vi "Create an FPGA Addon and selectively import scalars.vi"() -> ()   [LabVIEW 2018]
uses:
  <vilib>/addons/VeriStand Custom Device Scripting APIs/FPGA Addon/Scripting API.lvlibp/APIs/Scripting API/TypeDefs/Output Scalar Data.ctl
  <vilib>/addons/VeriStand Custom Device Scripting APIs/FPGA Addon/Scripting API.lvlibp/Addon/Addon Shared/Types/Data Type.ctl
  <vilib>/addons/VeriStand Custom Device Scripting APIs/FPGA Addon/Scripting API.lvlibp/APIs/Scripting API/TypeDefs/Input Scalar Data.ctl
  <vilib>/addons/VeriStand Custom Device Scripting APIs/FPGA Addon/Scripting API.lvlibp/APIs/Scripting API/Public/Bitfile Resources/Import Bitfile Scalars (Instances)/Import Scalars - by label.vi
  <vilib>/addons/VeriStand Custom Device Scripting APIs/FPGA Addon/Scripting API.lvlibp
  <vilib>/addons/VeriStand Custom Device Scripting APIs/FPGA Addon/Scripting API.lvlibp/Addon/Addon Shared/FPGA Addon Shared.lvlib
panel:
  out "imported bitfile scalars out":T1[](array[typedef])
  out "error out":errorcluster
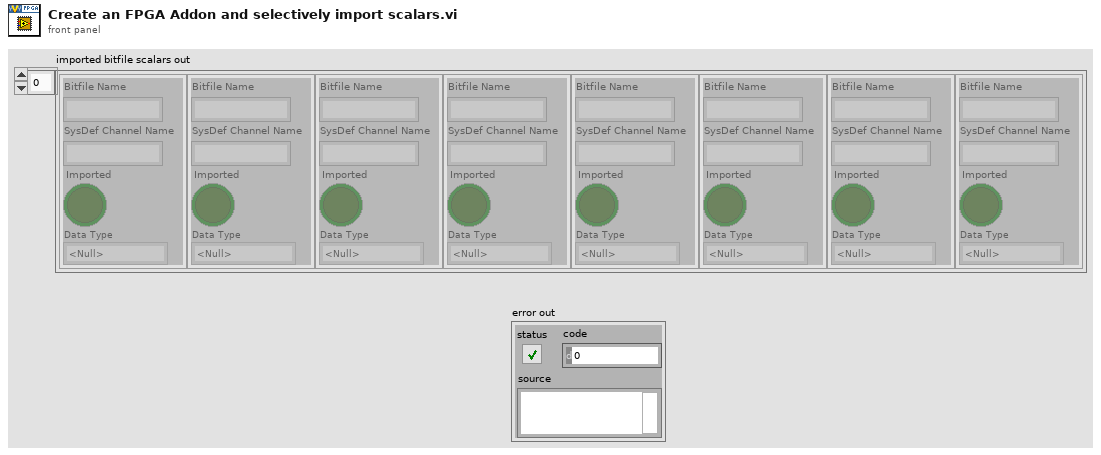
[diagram p1: front panel]
types:
  T1 = typedef "Scripting API.lvlibp/Output Scalar Data.ctl" = cluster{"Bitfile Name":string, "SysDef Channel Name":string, "Imported":bool, "Data Type":T2}
  T2 = typedef "Scripting API.lvlibp/FPGA Addon Shared.lvlib/Data Type.ctl" = enum8{"<Null>", "I8", "I16", "I32", "I64", "U8", "U16", "U32", "U64", "SGL", "Boolean", "Analog PWM In Settings", "Analog PWM In", "Digital PWM In Settings", "Digital PWM In", "Digital PWM Out", "Sine Out", "FXP+/-24.5", "FXP+/-16.5", "FXP+/-32.8", "FXP+/-64.32", "FXP+/-16.7", "FXP+/-20.5", "FXP+/-27.5", "FXP+/-32.16", "FXP+16.3", "FXP+18.3", "Digital Static In", "Digital Static Out", "Digital Static In Settings", "Digital WSS Out", "Quad Encoder Settings", "Quad Encoder In", "Group"}
  T3 = typedef "Scripting API.lvlibp/Input Scalar Data.ctl" = cluster{"Bitfile Name":string, "SysDef Name":string}
  T4 = typedef "Scripting API.lvlibp/Custom Device API.lvlib/Custom Device Item Ref.ctl" = u64
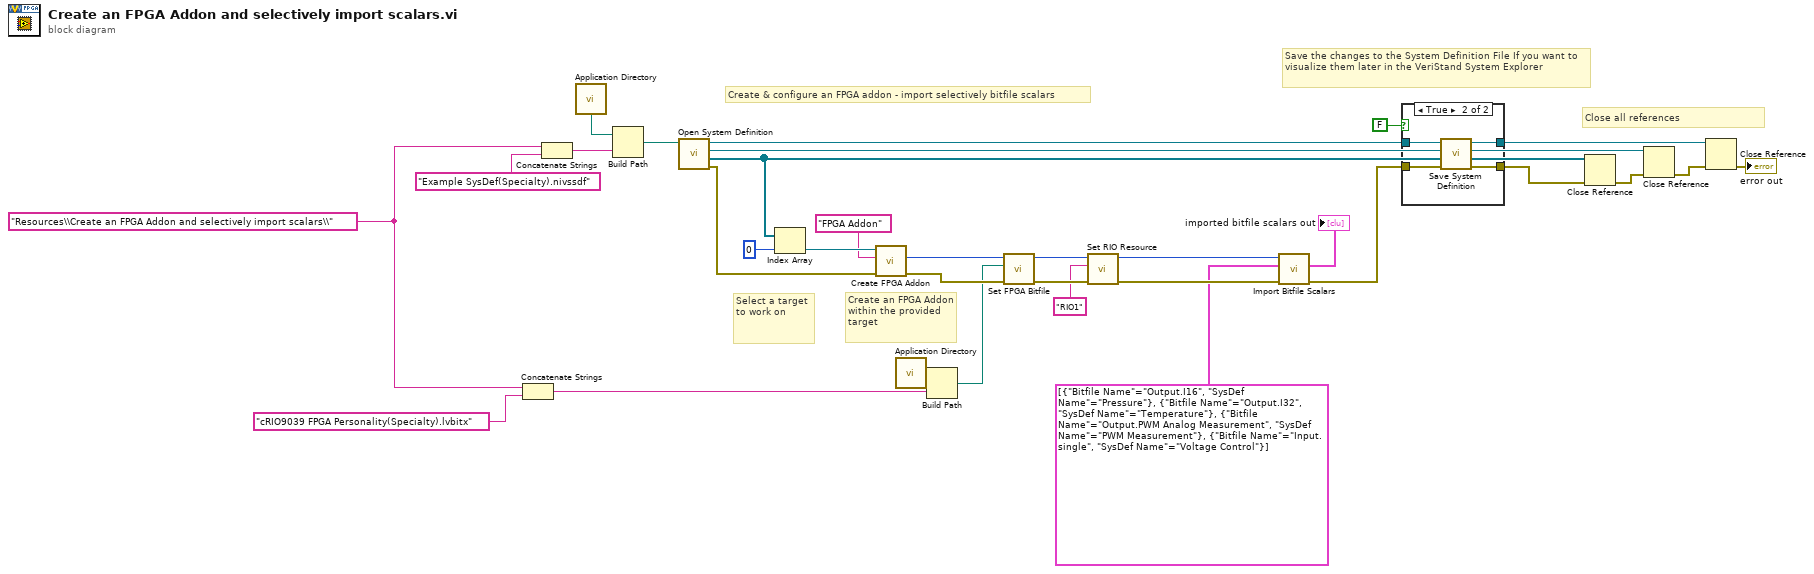
[diagram p0: block diagram]
diagram:
  w15 = "Resources\\Create an FPGA Addon and selectively import scalars\\" ("name or relative path")
  # "Create & configure an FPGA addon - import selectively bitfile scalars"
  # "Save the changes to the System Definition File If you want to visualize them later in the VeriStand System Explorer"
  # "Close all references"
  # "Create an FPGA Addon within the provided target"
  # "Select a target to work on"
  n1 = Concatenate Strings(w15, "cRIO9039 FPGA Personality(Specialty).lvbitx" ("name or relative path")) -> (w13:string)
  n2 = Concatenate Strings(w15, "Example SysDef(Specialty).nivssdf" ("name or relative path")) -> (w16:string)
  n3 = call <vilib>:"Application Directory.vi"() -> ("Application Directory"=w27:path)
  n4 = Build Path(base path=w27, name or relative path=w16) -> (appended path=w26:path)
  n5 = call "Open System Definition.vi"("System Definition File"=w26) -> ("error out"=w18:errorcluster, "targets refnums"=w30:refnum<k24>[], "root refnum"=w31:refnum<k24>, "system definition refnum"=w24:refnum<k24>)  [unwired: 7 in]
  n6 = Index Array(array=w30, index=0) -> (element=w20:refnum<k24>)
  n7 = call <vilib>:"Create FPGA Addon.vi"("error in"=w18, "FPGA addon name"="FPGA Addon" ("fpga addon name"), "target in"=w20) -> ("error out"=w11:errorcluster, "FPGA addon refnum"=w10:T4)  [unwired: 6 in, 1 out]
  n8 = call <vilib>:"Application Directory.vi"() -> ("Application Directory"=w21:path)
  n9 = Build Path(base path=w21, name or relative path=w13) -> (appended path=w9:path)
  n10 = call <vilib>:"Set FPGA Bitfile.vi"("error in"=w11, "FPGA bitfile path"=w9, "FPGA addon refnum in"=w10) -> ("error out"=w8:errorcluster, "FPGA addon refnum out"=w7:T4)  [unwired: 7 in]
  n11 = call <vilib>:"Set RIO Resource.vi"("error in"=w8, "RIO resource in"="RIO1", "FPGA addon refnum in"=w7) -> ("error out"=w5:errorcluster, "FPGA addon refnum out"=w4:T4)  [unwired: 7 in]
  n12 = call-poly <vilib>:"Import Bitfile Scalars.vi"("error in"=w5, "bitfile scalars in"=T3[] [{"Bitfile Name"="Output.I16", "SysDef Name"="Pressure"}, {"Bitfile Name"="Output.I32", "SysDef Name"="Temperature"}, {"Bitfile Name"="Output.PWM Analog Measurement", "SysDef Name"="PWM Measurement"}, {"Bitfile Name"="Input.single", "SysDef Name"="Voltage Control"}], "FPGA addon refnum in"=w4) -> ("error out"=w3:errorcluster, "imported bitfile scalars out"=→"imported bitfile scalars out":T1[])  [unwired: 6 in, 1 out]
  n13 = case shown="True" FALSE {
    tunnel: w24 -> [w34 w38]
    tunnel: [w34 w37] -> w23
    tunnel: [w33 w36] -> w22
    tunnel: w3 -> [w33 w35]
    frame False {
    }
    frame True {
      n14 = call "Save System Definition.vi"("error in (no error)"=w35, ".NET Refnum in"=w38) -> ("error out"=w36:errorcluster, ".NET Refnum out"=w37:refnum<k24>)  [unwired: 8 in]
    }
  }
  n15 = Close Reference(reference=w30, error in (no error)=w22) -> (error out=w29:errorcluster)
  n16 = Close Reference(reference=w31, error in (no error)=w29) -> (error out=w28:errorcluster)
  n17 = Close Reference(reference=w23, error in (no error)=w28) -> (error out=→"error out":errorcluster)
